vi "4xFFT.vi"(8 "Input 4":u16, 9 "Input 3":u16, 10 "Input 2":u16, 11 "Input 1":u16) -> (0 "real data out 4":fxp<+/-,23,8>, 1 "real data out 3":fxp<+/-,23,8>, 2 "real data out 2":fxp<+/-,23,8>, 3 "real data out":fxp<+/-,23,8>)   [LabVIEW 2020]
uses:
  <vilib>/rvi/Analysis/measure/FFT/simModelSupport/niFPGA FFT Outside SCTL Sim Properties.ctl
  <vilib>/rvi/Analysis/measure/FFT/simModelSupport/niFPGA FFT Sim Types.ctl
  <vilib>/rvi/Analysis/measure/FFT/simModelSupport/niFpgaFFTSimArithmeticProperties.ctl
  <vilib>/rvi/Analysis/measure/FFT/simModelSupport/niFpgaFFTSimDfxp.ctl
  <vilib>/fxp/LVFixedPointQuantizationPolicyTypeDef.ctl
  <vilib>/rvi/Emulation/niFpgaGetClockAttributes.vi
  <vilib>/rvi/Emulation/niFpgaSctlEmulationGetInTimedLoop.vi
  <vilib>/rvi/Emulation/niFpgaEmulationReportErrorSimple.vi
  <vilib>/rvi/Analysis/measure/FFT/simModelSupport/niFpgaFFTSimModelOutsideSCTLCore.vi
  <vilib>/rvi/Emulation/niFpgaCriticalErrorInLSC.vi
  <vilib>/rvi/FXPMathLib/FxpInterpret/XNode/nifxpmath_Interpret.xnode
  <vilib>/rvi/Analysis/measure/FFT/XNode/niFpgaFFT.xnode
panel:
  out "data index 4":u16
  out "data index 3":u16
  out "data index 2":u16
  out "data index":u16
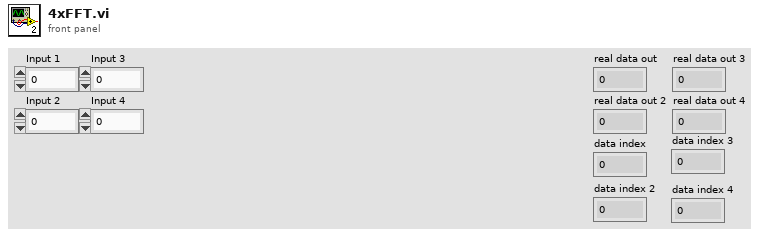
[diagram p1: front panel]
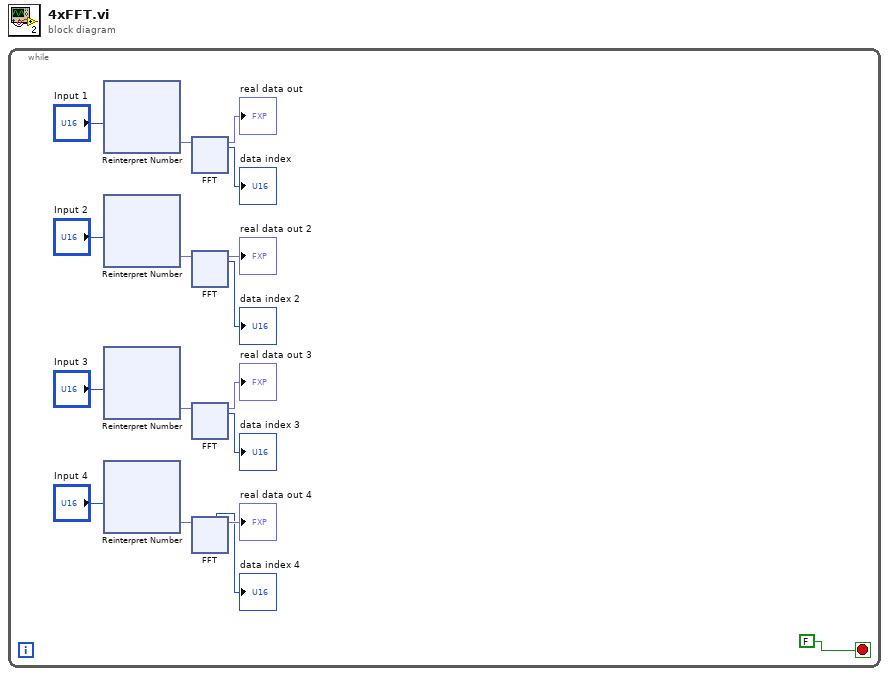
[diagram p0: block diagram]
diagram:
  n1 = while {
    stop <- FALSE stop-if-true
    n2 = xnode "Reinterpret Number"("x"="Input 1") -> ("y"=w15:fxp<+/-,16,1>)
    n3 = xnode "Reinterpret Number"("x"="Input 2") -> ("y"=w11:fxp<+/-,16,1>)
    n4 = xnode "Reinterpret Number"("x"="Input 3") -> ("y"=w10:fxp<+/-,16,1>)
    n5 = xnode "Reinterpret Number"("x"="Input 4") -> ("y"=w9:fxp<+/-,16,1>)
    n6 = xnode "FFT"("real data in"=w15) -> ("data index"=→"data index":u16, "real data out"=→"real data out":fxp<+/-,23,8>)  [unwired: 2 in, 2 out]
    n7 = xnode "FFT"("real data in"=w11) -> ("data index"=→"data index 2":u16, "real data out"=→"real data out 2":fxp<+/-,23,8>)  [unwired: 2 in, 2 out]
    n8 = xnode "FFT"("real data in"=w10) -> ("data index"=→"data index 3":u16, "real data out"=→"real data out 3":fxp<+/-,23,8>)  [unwired: 2 in, 2 out]
    n9 = xnode "FFT"("real data in"=w9) -> ("data index"=→"data index 4":u16, "real data out"=→"real data out 4":fxp<+/-,23,8>)  [unwired: 2 in, 2 out]
  }
